vi "UUID.vi"() -> (1 "UUIDlower":u64 format="%x", 2 "UUIDupper":u64 format="%x", 3 "UUID":string)   [LabVIEW 2014]
doc: "Generates a UUID per the IETF RFC-4122 specification, version 4.\n\n\nVersion 1.0 - 02/13/2013\n\nPhaeron, Inc.\nwww.phaeron.com\ninfo@phaeron.com"
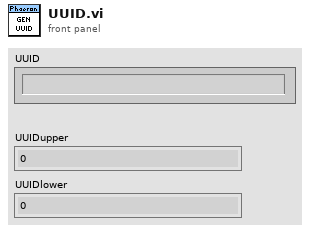
[diagram p1: front panel]
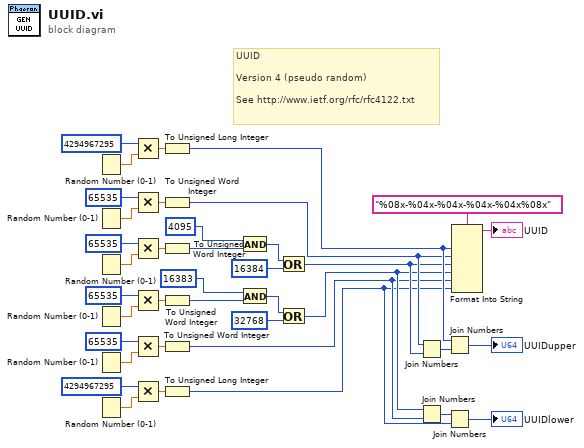
[diagram p0: block diagram]
diagram:
  # "UUID\n\nVersion 4 (pseudo random)\n\nSee http://www.ietf.org/rfc/rfc4122.txt"
  n1 = Random Number (0-1)() -> (number: 0 to 1=w37:dbl)
  n2 = Random Number (0-1)() -> (number: 0 to 1=w34:dbl)
  n3 = Random Number (0-1)() -> (number: 0 to 1=w15:dbl)
  n4 = Random Number (0-1)() -> (number: 0 to 1=w32:dbl)
  n5 = Random Number (0-1)() -> (number: 0 to 1=w26:dbl)
  n6 = Random Number (0-1)() -> (number: 0 to 1=w31:dbl)
  n7 = Multiply(x=u32 4294967295, y=w37) -> (x*y=w29:dbl)
  n8 = Multiply(x=u16 65535, y=w34) -> (x*y=w27:dbl)
  n9 = Multiply(x=u16 65535, y=w15) -> (x*y=w16:dbl)
  n10 = Multiply(x=u32 65535, y=w32) -> (x*y=w23:dbl)
  n11 = Multiply(x=u16 65535, y=w26) -> (x*y=w24:dbl)
  n12 = Multiply(x=u32 4294967295, y=w31) -> (x*y=w28:dbl)
  n13 = To Unsigned Long Integer(number=w29) -> (unsigned 32bit integer=w10:u32)
  n14 = To Unsigned Word Integer(number=w27) -> (unsigned 16bit integer=w7:u16)
  n15 = To Unsigned Word Integer(number=w16) -> (unsigned 16bit integer=w17:u16)
  n16 = To Unsigned Word Integer(number=w23) -> (unsigned 16bit integer=w12:u16)
  n17 = To Unsigned Word Integer(number=w24) -> (unsigned 16bit integer=w2:u16)
  n18 = To Unsigned Long Integer(number=w28) -> (unsigned 32bit integer=w1:u32)
  n19 = And(x=u16 4095, y=w17) -> (x .and. y?=w19:u16)
  n20 = And(x=u16 16383, y=w12) -> (x .and. y?=w21:u16)
  n21 = Or(x=w19, y=u16 16384) -> (x .or. y?=w6:u16)
  n22 = Or(x=w21, y=u16 32768) -> (x .or. y?=w3:u16)
  n23 = Join Numbers(hi=w7, lo=w6) -> ((hi.lo)=w9:u32)
  n24 = Join Numbers(hi=w3, lo=w2) -> ((hi.lo)=w4:u32)
  n25 = Join Numbers(hi=w10, lo=w9) -> ((hi.lo)=→"UUIDupper":u64)
  n26 = Join Numbers(hi=w4, lo=w1) -> ((hi.lo)=→"UUIDlower":u64)
  n27 = Format Into String(format string="%08x-%04x-%04x-%04x-%04x%08x", w10, w7, w6, w3, w2, w1) -> (resulting string=→"UUID":string)  [unwired: 2 in, 1 out]
